vi "SendToDb.vi"(8 "error in (no error)":errorcluster, 10 "Value DBL":dbl, 11 "AnalogComparator in":refnum<class "AbruptChange.lvclass">) -> (0 "error out":errorcluster, 3 "AnalogComparator out":refnum<class "AbruptChange.lvclass">)   [LabVIEW 2019, in "AbruptChange.lvclass"]
uses:
  AbruptChange.lvclass
  D:/GIT H4000/H4000/src/Proccess_class/Proccess.lvclass
  Logger_class/EventData.ctl
  TypeDef/AlarmType.ctl
  Proccess_class/Proccess.lvclass/Proccess.ctl
  AbruptChange.lvclass/AbruptChange.ctl
  Logger_class/Logger.lvclass
  Proccess_class/Proccess.lvclass
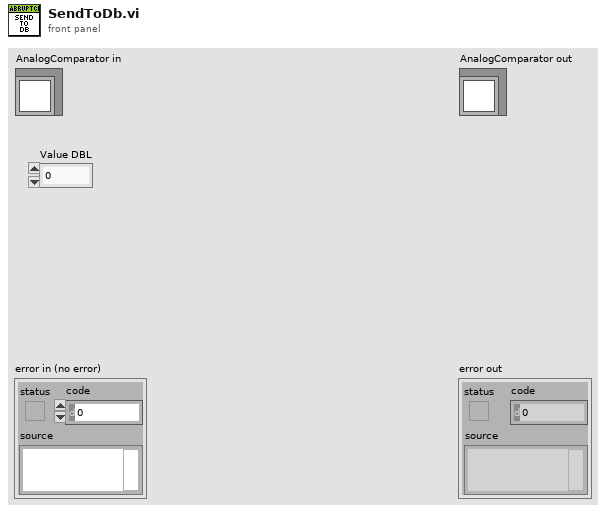
[diagram p1: front panel]
types:
  T1 = typedef "AlarmType.ctl" = enum16{"Normal", "Warning", "Alarm"}
  T2 = typedef "EventData.ctl" = cluster{"obj_tag":string, "event_tag":string, "Description":string, "ALARM TYPE":T1, "Value DBL":dbl, "Value INT":i32, "Value STR":string, "Time Stamp":timestamp}
  T3 = typedef "Proccess.lvclass/TAGs.ctl" = cluster{"TAG":string, "PTAG":string, "DESC":string}
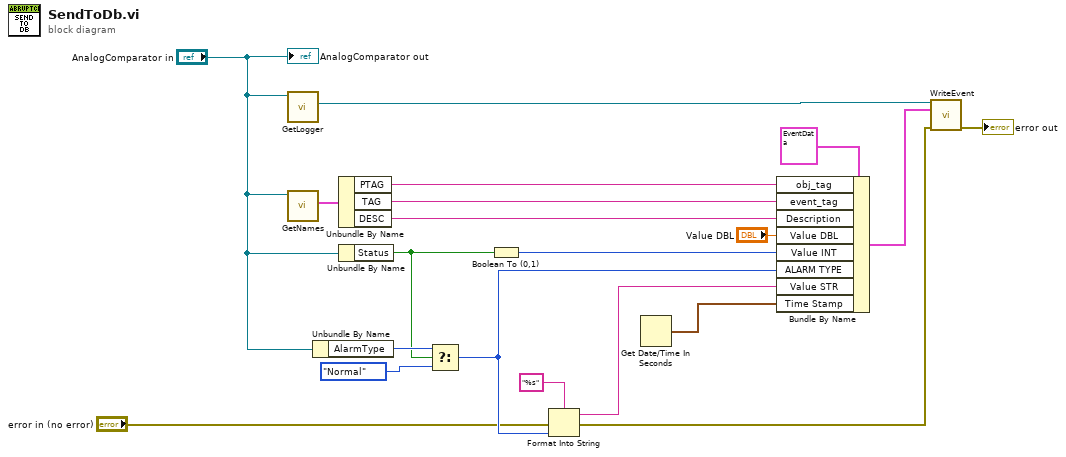
[diagram p0: block diagram]
diagram:
  n1 = call "GetLogger.vi"("Proccess in"="AnalogComparator in") -> ("Logger"=w18:refnum<class "Logger.lvclass">)  [unwired: 10 in]
  n2 = call "GetNames.vi"("Proccess in"="AnalogComparator in") -> ("Tags"=w17:T3)  [unwired: 10 in]
  n3 = Unbundle By Name("AnalogComparator in") -> ("AlarmType"=w11:T1)
  n4 = Unbundle By Name(w17) -> ("PTAG"=w15:string, "TAG"=w14:string, "DESC"=w13:string)
  n5 = Unbundle By Name("AnalogComparator in") -> ("Status"=w10:bool)
  n6 = Select(t=w11, s=w10, f=AlarmType."Normal") -> (s? t:f=w6:T1)
  n7 = Boolean To (0,1)(Boolean=w10) -> (0, 1=w12:i16)
  n8 = Format Into String(format string="%s", error in="error in (no error)", w6) -> (resulting string=w7:string, error out=w2:errorcluster)  [unwired: 1 in]
  n9 = Get Date/Time In Seconds() -> (seconds since 1Jan1904=w5:timestamp)
  n10 = Bundle By Name(cluster=T2 {"obj_tag"="", "event_tag"="", "Description"="", "ALARM TYPE"=enum."Alarm", "Value DBL"=0.0, "Value INT"=0, "Value STR"="", "Time Stamp"=timestamp(0 s since 1904-01-01)} ("Event"), "obj_tag"=w15, "event_tag"=w14, "Description"=w13, "Value DBL"="Value DBL", "Value INT"=w12, "ALARM TYPE"=w6, "Value STR"=w7, "Time Stamp"=w5) -> (w3:T2)
  n11 = call "WriteEvent.vi"("reference in"=w18, "Event"=w3, "error in (no error)"=w2) -> ("error out"=→"error out":errorcluster)  [unwired: 11 in, 1 out]
  "AnalogComparator out" <- "AnalogComparator in"
